vi "SSC Relay Control Multiple Actions Per-Relay Pin.vi"(0 "SSC Relay in":T1[](array[typedef]), 1 "Wait Between Relays (s)":dbl, 5 "Relay Actions":T3[](array[typedef]) items=["Open Relay"=20, "Close Relay"=21], 7 "Settling Time (s)":dbl format="%#_12p", 9 "Relay Pins":string[](array[string]), 11 "error in":errorcluster) -> (4 "SSC Relay out":T1[](array[typedef]), 8 "Completed Relay Operations":T2[](array[typedef]) {"Desired State" items=["Open Relay"=20, "Close Relay"=21]}, 15 "error out":errorcluster)   [LabVIEW 2019]
doc: "Performs the specified relay action for each Relays configured in the SSC Relay session, one Relay at a time. The function will then wait a specified amount of time if the Settling Time (s) input is wired. \n\nThere must be at exactly one Relay Action per Relay configured in the SSC Relay session, otherwise the function will return an error. \n\nUse the Wait Between Relay (s) input if a wait time is desired between relay actions."
uses:
  SSC Relay.ctl
  <instrlib>/niSwitch/niSwitch.llb/niSwitch Relay Action.ctl
  SubVIs/TSM Relay Completed Operations.ctl
  SSC Relay Control Core.vi
  Single SSC Relay NI-Switch Control.vi
  Single SSC Relay Fill Additional Error info.vi
  SSC Relay Expand Action Array to All Sessions.vi
  <instrlib>/niSwitch/niSwitch.llb/niSwitch Get Relay Position.vi
  <instrlib>/niSwitch/niSwitch.llb/niSwitch Relay Control.vi
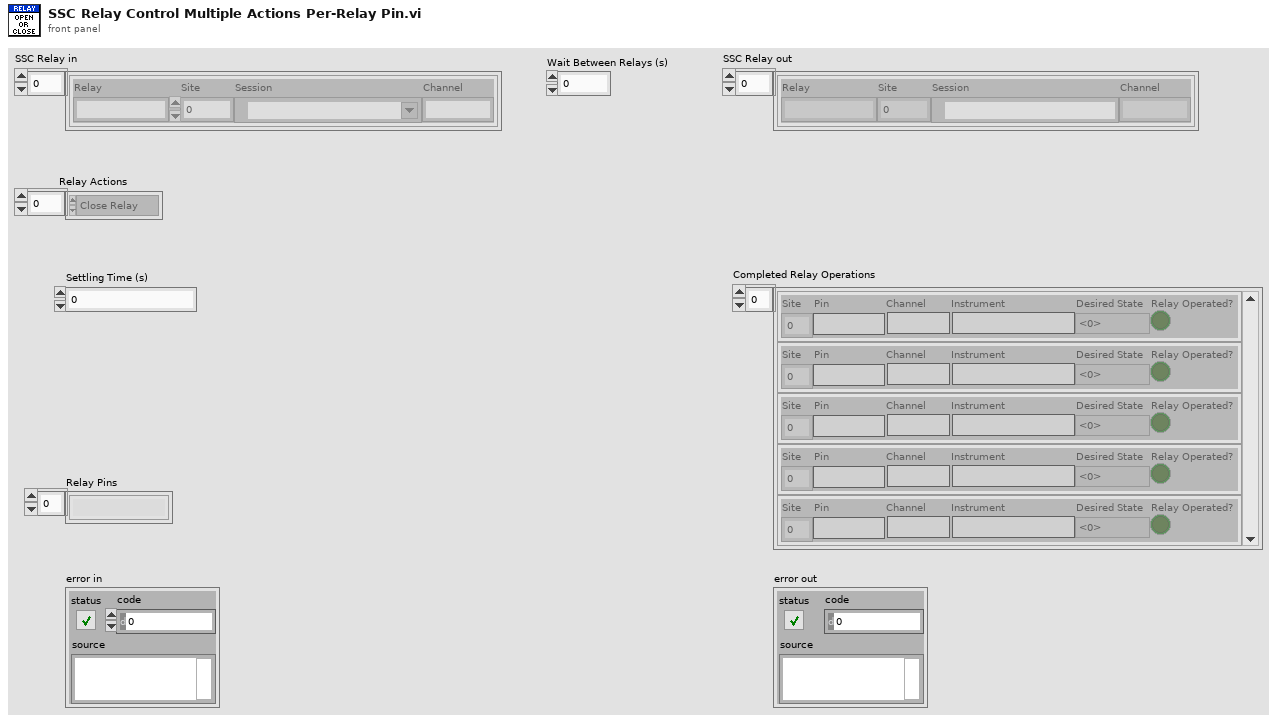
[diagram p1: front panel]
types:
  T1 = typedef "SSC Relay.ctl" = cluster{"Relay":string, "Site":i32, "Session":refnum<k15>, "Channel":string}
  T2 = typedef "TSM Relay Completed Operations.ctl" = cluster{"Site":i32, "Pin":string, "Channel":string, "Instrument":string, "Desired State":T3, "Relay Operated?":bool}
  T3 = typedef "niSwitch Relay Action.ctl" = i32
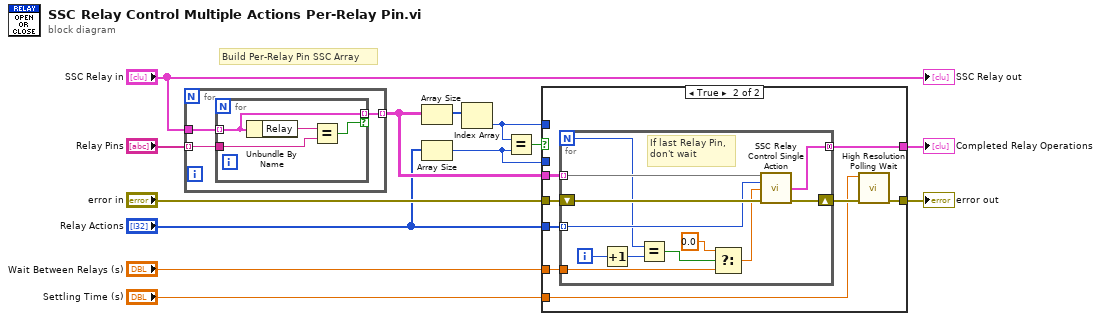
[diagram p0: block diagram]
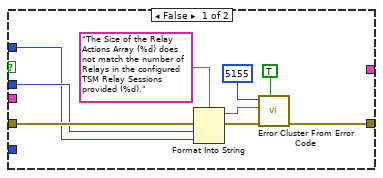
[diagram p2: hidden frame]
diagram:
  # "Build Per-Relay Pin SSC Array"
  n1 = for {
    tunnel: "SSC Relay in" -> [w16]
    tunnel: [w15] -> w4 mode=indexing
    tunnel: "Relay Pins" -> [w14] mode=indexing
    n2 = for {
      tunnel: w16 -> [w20] mode=indexing
      tunnel: [w20] -> w15 mode=indexing if=w18
      tunnel: w14 -> [w17]
      n3 = Unbundle By Name(w20) -> ("Relay"=w19:string)
      n4 = Equal?(x=w19, y=w17) -> (x = y?=w18:bool)
    }
  }
  n5 = Array Size(array=w4) -> (size(s)=w13:i32[])
  n6 = Array Size(array="Relay Actions") -> (size(s)=w10:i32)
  n7 = Index Array(array=w13) -> (element=w11:i32)  [unwired: 1 in]
  n8 = Equal?(x=w11, y=w10) -> (x = y?=w12:bool)
  n9 = case shown="True" w12 {
    tunnel: [w26 w37] -> w6
    tunnel: "Wait Between Relays (s)" -> [_ w36]
    tunnel: "error in" -> [w27 w35]
    tunnel: [_ w34] -> w5
    tunnel: "Settling Time (s)" -> [_ w32]
    tunnel: w4 -> [_ w31]
    tunnel: "Relay Actions" -> [_ w30]
    tunnel: w11 -> [w21 _]
    tunnel: w10 -> [w22 _]
    frame False {
      n10 = Format Into String(format string="The Size of the Relay Actions Array (%d) does not match the number of Relays in the configured TSM Relay Sessions provided (%d)." ("error message (\"\")"), error in=w27, w22, w21) -> (resulting string=w23:string, error out=w25:errorcluster)  [unwired: 1 in]
      n11 = call <vilib>:"Error Cluster From Error Code.vi"("show call chain? (False)"=TRUE, "error in (no error)"=w25, "error message (\"\")"=w23, "error code (0)"=5155) -> ("error out"=w26:errorcluster)  [unwired: 5 in]
    }
    frame True {
      n12 = for {
        N -> [w39]
        tunnel: w36 -> [w47]
        tunnel: w31 -> [w40] mode=indexing
        tunnel: [w38] -> w34 mode=concatenating
        tunnel: w30 -> [w41] mode=indexing
        shift-right: [w43] -> w33
        shift-left: w35 -> [w44]
        i -> [w49]
        # "If last Relay Pin, don't wait"
        n13 = Increment(x=w49) -> (x+1=w45:i32)
        n14 = Equal?(x=w39, y=w45) -> (x = y?=w48:bool)
        n15 = Select(t=0.0, s=w48, f=w47) -> (s? t:f=w42:dbl)
        n16 = call "SSC Relay Control Single Action.vi"("SSC Relay in"=w40, "Relay Action"=w41, "Settling Time (s)"=w42, "error in"=w44) -> ("Completed Relay Operations"=w38:T2[], "error out"=w43:errorcluster)  [unwired: 9 in, 1 out]
      }
      n17 = call <vilib>:"High Resolution Polling Wait.vi"("error in (no error)"=w33, "seconds to wait"=w32) -> ("error out"=w37:errorcluster)  [unwired: 9 in]
    }
  }
  "error out" <- w6
  "Completed Relay Operations" <- w5
  "SSC Relay out" <- "SSC Relay in"
